vi "DSF.Engine.Runtime.Plugin.Create.vi"(5 "id":i32, 7 "Timing":refnum<class "DSF.Engine.Timing.lvclass">, 8 "error in (no error)":errorcluster, 9 "Plugin Cache":refnum<class "DSF.Engine.Memory.Cache.Plugin.lvclass">, 10 "Plugin Interface":refnum<class "DSF.Engine.Interface.Plugin.lvclass">, 11 "Plugin Runtime in":refnum<class "DSF.Engine.Runtime.Plugin.lvclass">) -> (0 "error out":errorcluster, 3 "Plugin Runtime out":refnum<class "DSF.Engine.Runtime.Plugin.lvclass">)   [LabVIEW 2016, in "DSF.Engine.lvlib" / "DSF.Engine.Runtime.Plugin.lvclass"]
uses:
  DSF.Engine.Runtime.Plugin.lvclass
  C:/Git/Sourcetree/DSF/Source/Engine/Classes/Runtime/DSF.Engine.Runtime.lvclass
  Timing/DSF.Engine.Timing.lvclass
  Interface/DSF.Engine.Interface.Plugin.lvclass
  Cache/DSF.Engine.Memory.Cache.Plugin.lvclass
  DSF.Engine.Runtime.Plugin.lvclass/DSF.Engine.Runtime.Plugin.ctl
  Runtime/DSF.Engine.Runtime.lvclass
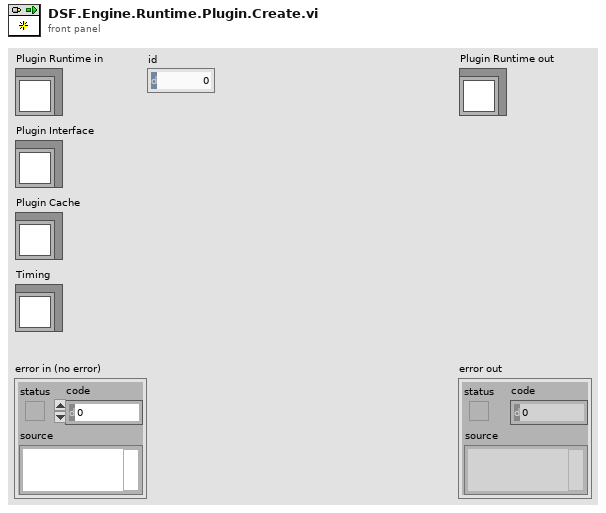
[diagram p1: front panel]
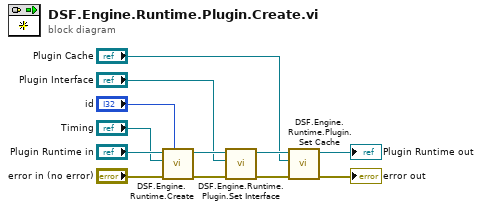
[diagram p0: block diagram]
diagram:
  n1 = call "DSF.Engine.Runtime.Create.vi"("id"="id", "error in (no error)"="error in (no error)", "Timing"="Timing", "DSF Runtime in"="Plugin Runtime in") -> ("error out"=w9:errorcluster, "DSF Runtime out"=w8:refnum<class "DSF.Engine.Runtime.Plugin.lvclass">)  [unwired: 6 in]
  n2 = call "DSF.Engine.Runtime.Plugin.Set Interface.vi"("error in (no error)"=w9, "Plugin Interface"="Plugin Interface", "Plugin Runtime in"=w8) -> ("error out"=w7:errorcluster, "Plugin Runtime out"=w4:refnum<class "DSF.Engine.Runtime.Plugin.lvclass">)  [unwired: 7 in]
  n3 = call "DSF.Engine.Runtime.Plugin.Set Cache.vi"("error in (no error)"=w7, "Plugin Cache"="Plugin Cache", "Plugin Runtime in"=w4) -> ("error out"=→"error out":errorcluster, "Plugin Runtime out"=→"Plugin Runtime out":refnum<class "DSF.Engine.Runtime.Plugin.lvclass">)  [unwired: 7 in]
